vi "10.vi"() -> ()   [LabVIEW 2023]
uses:
  <vilib>/Analysis/baseanly.llb/Mean (DBL).vi
  <vilib>/Utility/file.llb/Read Delimited Spreadsheet (string).vi
  <vilib>/Analysis/NI_AALBase.lvlib
panel:
  in  "OK Button 2":bool
  out "Waveform Graph":i32[](graph)
  out "Item Names":string[](array[string])
  in  "Listbox":i32(listbox)
  out "Array":string[](array[string])
  out "nume":string[](array[string])
  out "numere":string[][](array[string])
  in  "file path (dialog if empty)":path
  out "Table Control":string[][](table)
  in  "OK Button":bool
  in  "stop":bool
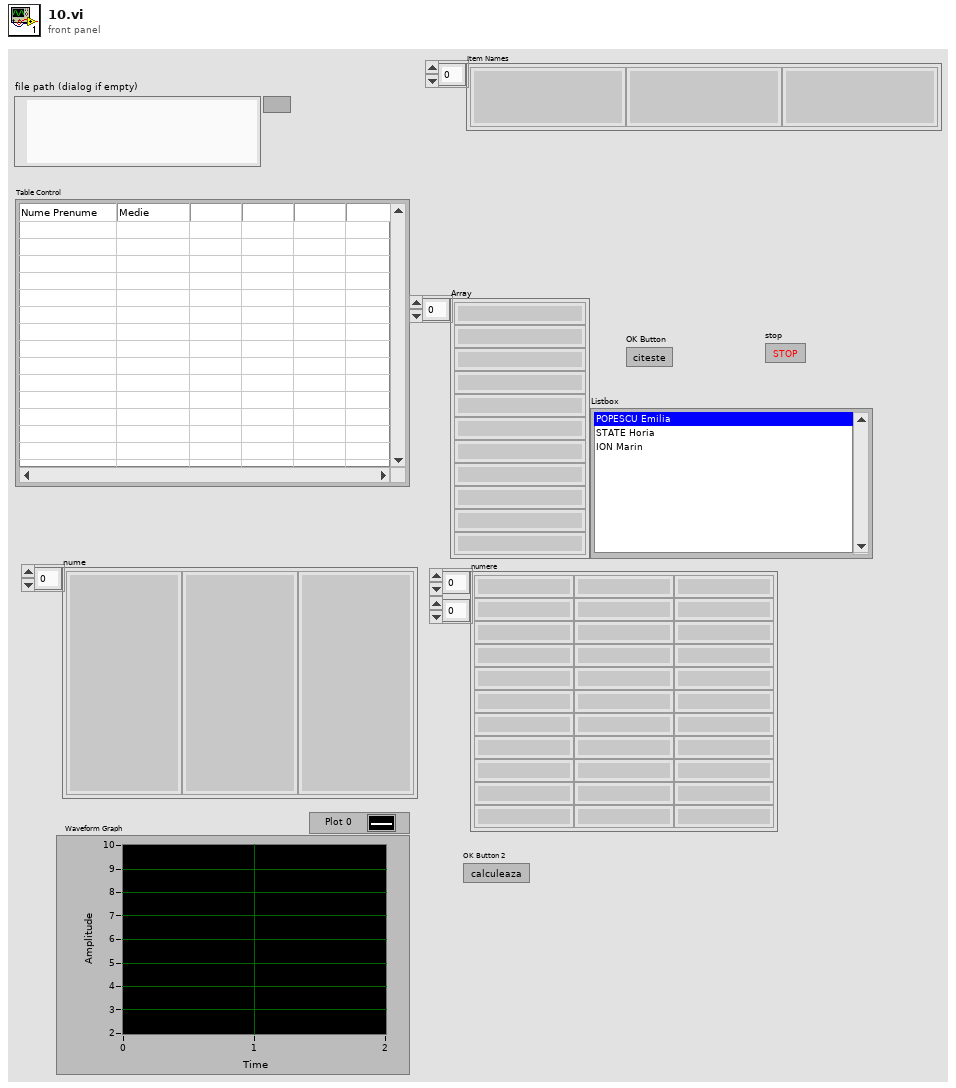
[diagram p1: front panel]
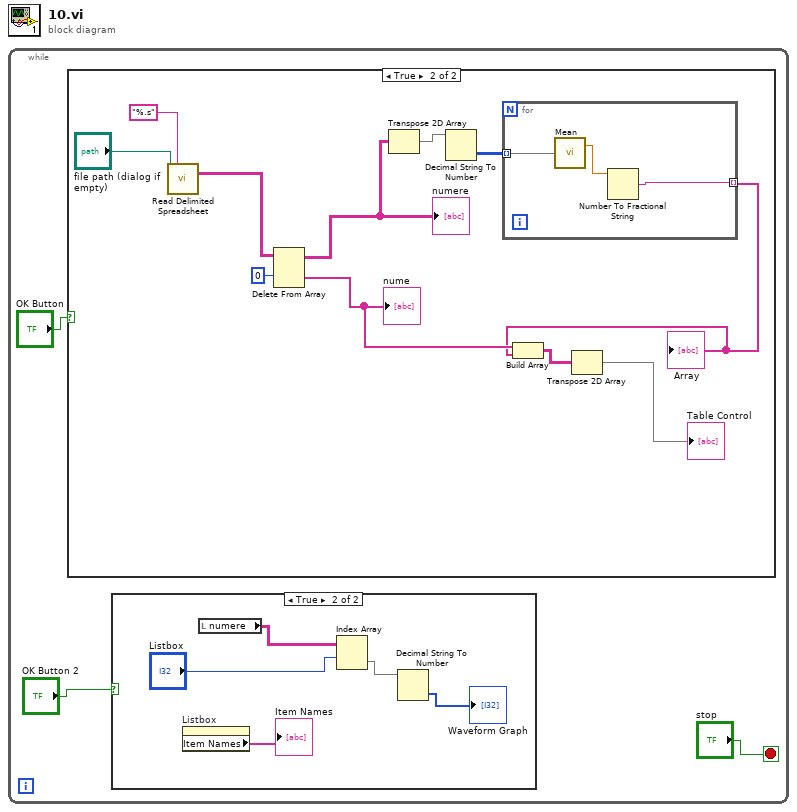
[diagram p0: block diagram]
diagram:
  n1 = while {
    stop <- "stop" stop-if-true
    n2 = case shown="True" "OK Button" {
      frame False {
      }
      frame True {
        n3 = call-poly <vilib>:"Read Delimited Spreadsheet.vi"("file path (dialog if empty)"="file path (dialog if empty)", "format (%s)"="%.s" ("format (%.3f)")) -> ("all rows"=w17:string[][])  [unwired: 8 in, 5 out]
        n4 = Delete From Array "Delete From Array"(array=w17, index (row)=0) -> (deleted portion=w13:string[], array with subset deleted=w9:string[][])  [unwired: 2 in]
        "numere" <- w9
        "nume" <- w13
        n5 = Transpose 2D Array(2D array=w9) -> (transposed array=w14:string[][])
        n6 = Decimal String To Number(string=w14) -> (number=w15:i32[][])  [unwired: 2 in, 1 out]
        n7 = for {
          tunnel: w15 -> [w22] mode=indexing
          tunnel: [w20] -> w10 mode=indexing
          n8 = call-poly <vilib>:"Mean.vi"("X"=w22) -> ("mean"=w21:dbl)  [unwired: 1 out]
          n9 = Number To Fractional String(number=w21) -> (F-format string=w20:string)  [unwired: 3 in]
        }
        "Array" <- w10
        n10 = Build Array(w13, w10) -> (w12:string[][])
        n11 = Transpose 2D Array(2D array=w12) -> (transposed array=→"Table Control":string[][])
      }
    }
    n12 = case shown="True" "OK Button 2" {
      frame False {
      }
      frame True {
        n13 = property on="Listbox" class="LstBox (strict)"() -> ("Item Names"=→"Item Names":string[])  [unwired: 2 in, 2 out]
        n14 = local read "numere"() -> (w4:string[][])
        n15 = Index Array "Index Array"(array=w4, index (row)="Listbox") -> (element=w7:string[])  [unwired: 1 in]
        n16 = Decimal String To Number(string=w7) -> (number=→"Waveform Graph":i32[])  [unwired: 2 in, 1 out]
      }
    }
  }
